vi "Run Service.vi"() -> ()   [LabVIEW 2023, in "BLSClimateChamberTemplateService_server.lvlib"]
uses:
  BLSClimateChamberTemplateService_server.lvlib
  <vilib>/gRPC/LabVIEW gRPC Servicer/ServiceBase/ServiceBase.lvclass
  <vilib>/gRPC/LabVIEW gRPC Servicer/Servicer/Servicer.lvclass/Servicer.ctl
  <vilib>/gRPC/LabVIEW gRPC Servicer/Servicer/Servicer.lvclass
panel:
  in  "Async [T] / Sync [F]":bool
  out "Listening Port":i32
  in  "Stop":bool
  in  "Server Address":string="localhost:50051"
  in  "Server Certificate File (.crt)":path
  in  "Server Key File (.key)":path
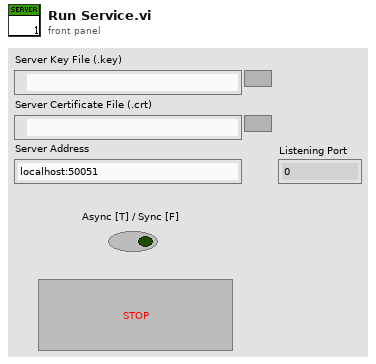
[diagram p1: front panel]
types:
  T1 = typedef "grpc-lvsupport-release.lvlib/grpcId.ctl" = u64
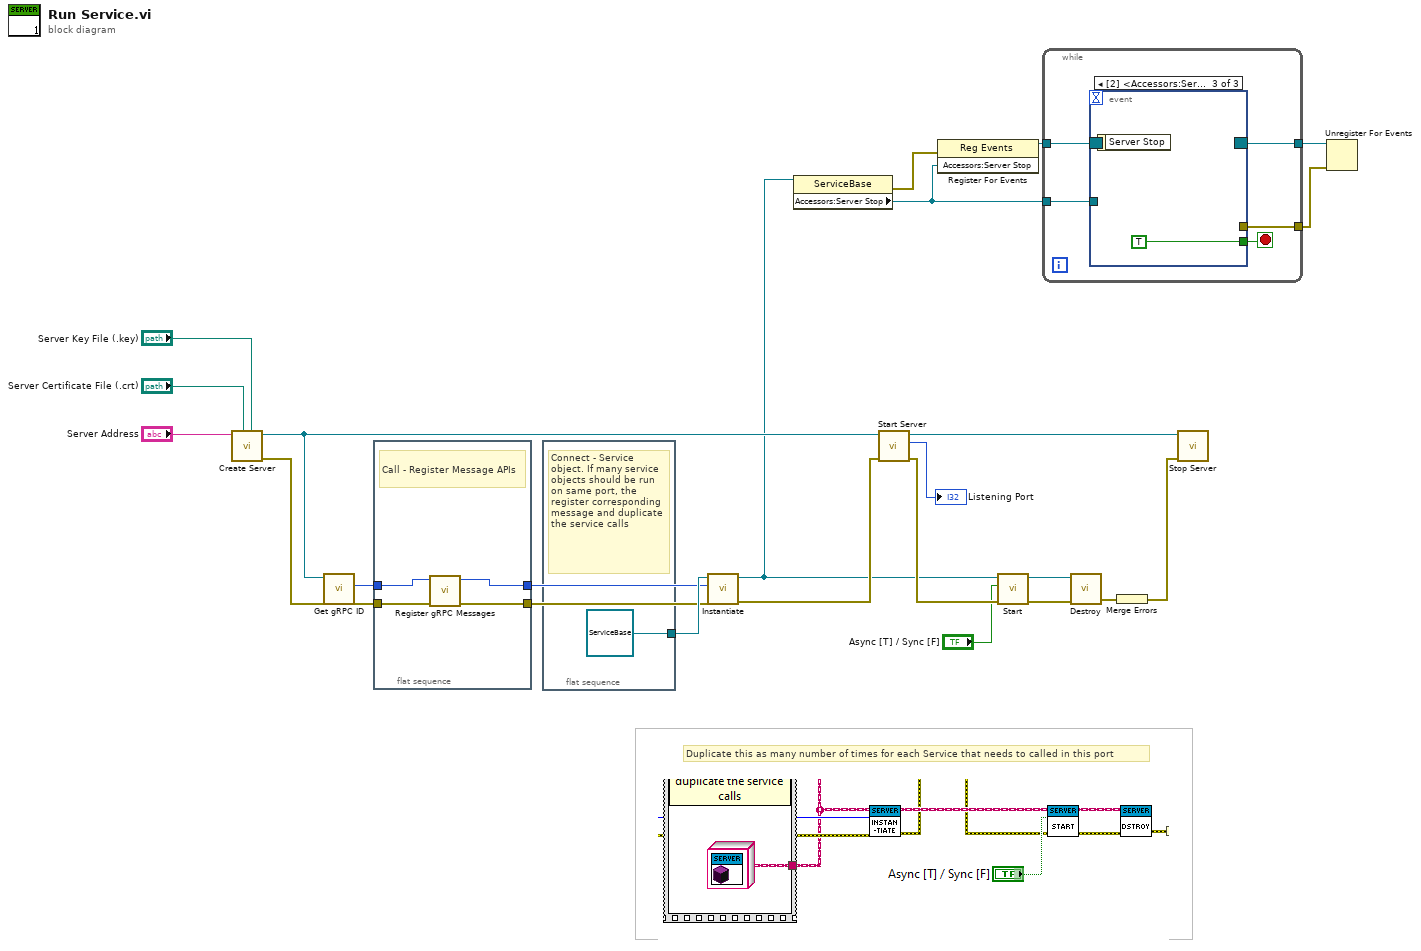
[diagram p0: block diagram]
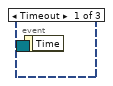
[diagram p2: hidden frame]
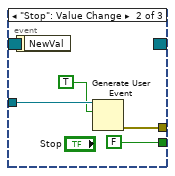
[diagram p3: hidden frame]
diagram:
  # "Duplicate this as many number of times for each Service that needs to called in this port"
  n1 = call <vilib>:"Create Server.vi"("Server Key File (.key)"="Server Key File (.key)", "Server Certificate File (.crt)"="Server Certificate File (.crt)", "Server Address"="Server Address") -> ("error out"=w9:errorcluster, "gRPC Server out"=w17:refnum<class "Servicer.lvclass">)  [unwired: 7 in]
  n2 = call <vilib>:"Get gRPC ID.vi"("OOP Server in"=w17) -> ("gRPC ID"=w10:T1)  [unwired: 9 in, 1 out]
  n3 = flat-sequence {
    tunnel: w10 -> [w26]
    tunnel: w9 -> [w28]
    tunnel: [w27] -> w8
    tunnel: [w25] -> w7
    frame #0 {
      # "Call - Register Message APIs"
      n4 = call "Register gRPC Messages.vi"("error in (no error)"=w28, "gRPC ID"=w26) -> ("error out"=w27:errorcluster, "gRPC ID Out"=w25:T1)  [unwired: 8 in]
    }
  }
  n5 = flat-sequence {
    tunnel: [refnum<class "ServiceBase.lvclass"> refnum ("gRPC-servicer.lvlib:iService.lvclass")] -> w11
    frame #0 {
      # "Connect - Service object. If many service objects should be run on same port, the register corresponding message and duplicate the service calls"
    }
  }
  n6 = call-dynamic "Instantiate.vi"("error in"=w8, "gRPCid"=w7, "iService"=w11) -> ("error out"=w15:errorcluster, "iService"=w2:refnum<class "ServiceBase.lvclass">)  [unwired: 7 in]
  n7 = property class="ServiceBase"(reference=w2) -> (error out=w16:errorcluster, "Accessors:Server Stop"=w1:refnum<user-event>)  [unwired: 1 in, 1 out]
  n8 = call <vilib>:"Start Server.vi"("error in"=w15, "gRPC Server in"=w17) -> ("error out"=w6:errorcluster, "Listening Port"=→"Listening Port":i32, "gRPC Server out"=w24:refnum<class "Servicer.lvclass">)  [unwired: 7 in]
  n9 = register-events(error in=w16, w1) -> (reference out=w20:refnum<event-registration>)  [unwired: 1 in, 1 out]
  n10 = call-dynamic "Start.vi"("error in"=w6, "ASync [T]"="Async [T] / Sync [F]", "iService in"=w2) -> ("error out"=w5:errorcluster, "iService out"=w4:refnum<class "ServiceBase.lvclass">)  [unwired: 7 in]
  n11 = while {
    tunnel: w20 -> [w34]
    tunnel: [w32] -> w19
    tunnel: [w30] -> w12
    tunnel: w1 -> [w31]
    stop <- w33 stop-if-true
    n12 = event shown="[2] <Accessors:Server Stop>: User Event" {
      selector: w34 -> [_ _ _]
      dyn-events: [_ _ _] -> w32
      timeout: _ -> [_ _ _]
      tunnel: [_ FALSE TRUE] -> w33
      tunnel: w31 -> [_ w37 _]
      tunnel: [_ w35 _] -> w30
      event Timeout {
        n13 = event-data() -> ()  [unwired: 1 in, 1 out]
      }
      event "Stop": Value Change {
        n14 = event-data() -> ()  [unwired: 1 in, 1 out]
        n15 = Generate User Event(user event=w37, event data cluster=TRUE ("event data")) -> (error out=w35:errorcluster)  [unwired: 2 in, 1 out]
      }
      event User Event {
        n16 = event-data() -> ()  [unwired: 1 in, 1 out]
      }
    }
  }
  n17 = call-dynamic "Destroy.vi"("error in"=w5, "SignalGeneratorService in"=w4) -> ("error out"=w14:errorcluster)  [unwired: 8 in, 1 out]
  n18 = Merge Errors(w14) -> (w13:errorcluster)
  n19 = call <vilib>:"Stop Server.vi"("error in"=w13, "gRPC Server in"=w24) -> ()  [unwired: 9 in, 1 out]
  n20 = Unregister For Events(event registration refnum=w19, error in=w12) -> ()  [unwired: 1 out]
